vi "队列采集速度.vi"() -> ()   [LabVIEW 2019, in "test.lvlib"]
uses:
  SubVI/test.lvlib
  SubVI/config.ctl
  <vilib>/NI/Modbus Library/API/Master/Modbus Master.lvclass
  SubVI/Instrument.ctl
  lib/QDInstrument.dll
panel:
  out "元素":T1={"initialize"="", "6221"={"6221 Resource"="GPIB0::24::INSTR", "Delta status"=FALSE}, "7001"={"Ch"=FALSE}, "SR830+6221"={"source"=0, "阻抗"=0.0, "量程入 4"=0, "量程入 3"=0, "量程入 2"=0, "量程入 1"=0, "电流"=0.0, "SR830 2"=FALSE, "SR830 3"=FALSE, "SR830 4"=FALSE, "SR830 1"=FALSE, "VISA 1"="", "VISA 2"="", "VISA 3"="", "VISA 4"="", "量程"=enum."量程每次测量会判定"}, "2400"={"2400"=FALSE, "VISA"=""}, "ch"={"ch str"="", "ch1"=FALSE, "ch2"=FALSE, "布尔"=FALSE}, "error"=FALSE, "数据文件路径"=path "", "log"={"log路径"=path "", "log interval"=0.0}, "Instrument"={"335 Resource"="GPIB0::24::INSTR", "Input (0:A)"=0, "Instrument Type"=3, "quantum design"=refnum, "Heater Output (1:1)"=1, "335state"=refnum, "semaphore"=refnum, "TCP master instance"=refnum}} {"Instrument"."Input (0:A)" items=["A", "B"]; "Instrument"."Instrument Type" items=["PPMS", "VersaLab", "DynaCool", "SVSM", "Lakeshore335", "PPMS-Rotate"]; "Instrument"."Heater Output (1:1)" items=["1"=1, "2"=2]; "SR830+6221"."source" items=["SR830 1", "SR830 2", "SR830 3", "SR830 4"]}
  out "簇":T1={"initialize"="", "6221"={"6221 Resource"="GPIB0::24::INSTR", "Delta status"=FALSE}, "7001"={"Ch"=FALSE}, "SR830+6221"={"source"=0, "阻抗"=0.0, "量程入 4"=0, "量程入 3"=0, "量程入 2"=0, "量程入 1"=0, "电流"=0.0, "SR830 2"=FALSE, "SR830 3"=FALSE, "SR830 4"=FALSE, "SR830 1"=FALSE, "VISA 1"="", "VISA 2"="", "VISA 3"="", "VISA 4"="", "量程"=enum."量程每次测量会判定"}, "2400"={"2400"=FALSE, "VISA"=""}, "ch"={"ch str"="", "ch1"=FALSE, "ch2"=FALSE, "布尔"=FALSE}, "error"=FALSE, "数据文件路径"=path "", "log"={"log路径"=path "", "log interval"=0.0}, "Instrument"={"335 Resource"="GPIB0::24::INSTR", "Input (0:A)"=0, "Instrument Type"=3, "quantum design"=refnum, "Heater Output (1:1)"=1, "335state"=refnum, "semaphore"=refnum, "TCP master instance"=refnum}} {"Instrument"."Input (0:A)" items=["A", "B"]; "Instrument"."Instrument Type" items=["PPMS", "VersaLab", "DynaCool", "SVSM", "Lakeshore335", "PPMS-Rotate"]; "Instrument"."Heater Output (1:1)" items=["1"=1, "2"=2]; "SR830+6221"."source" items=["SR830 1", "SR830 2", "SR830 3", "SR830 4"]}
  out "当前时间 4":timestamp
  out "数值 4":i32
  out "当前时间 3":timestamp
  out "数值 3":i32
  out "当前时间 2":timestamp
  out "数值 2":i32
  out "数值":i32
  out "当前时间":timestamp
  # "(真是通道1，假是通道2)"
  # "(真是通道1，假是通道2)"
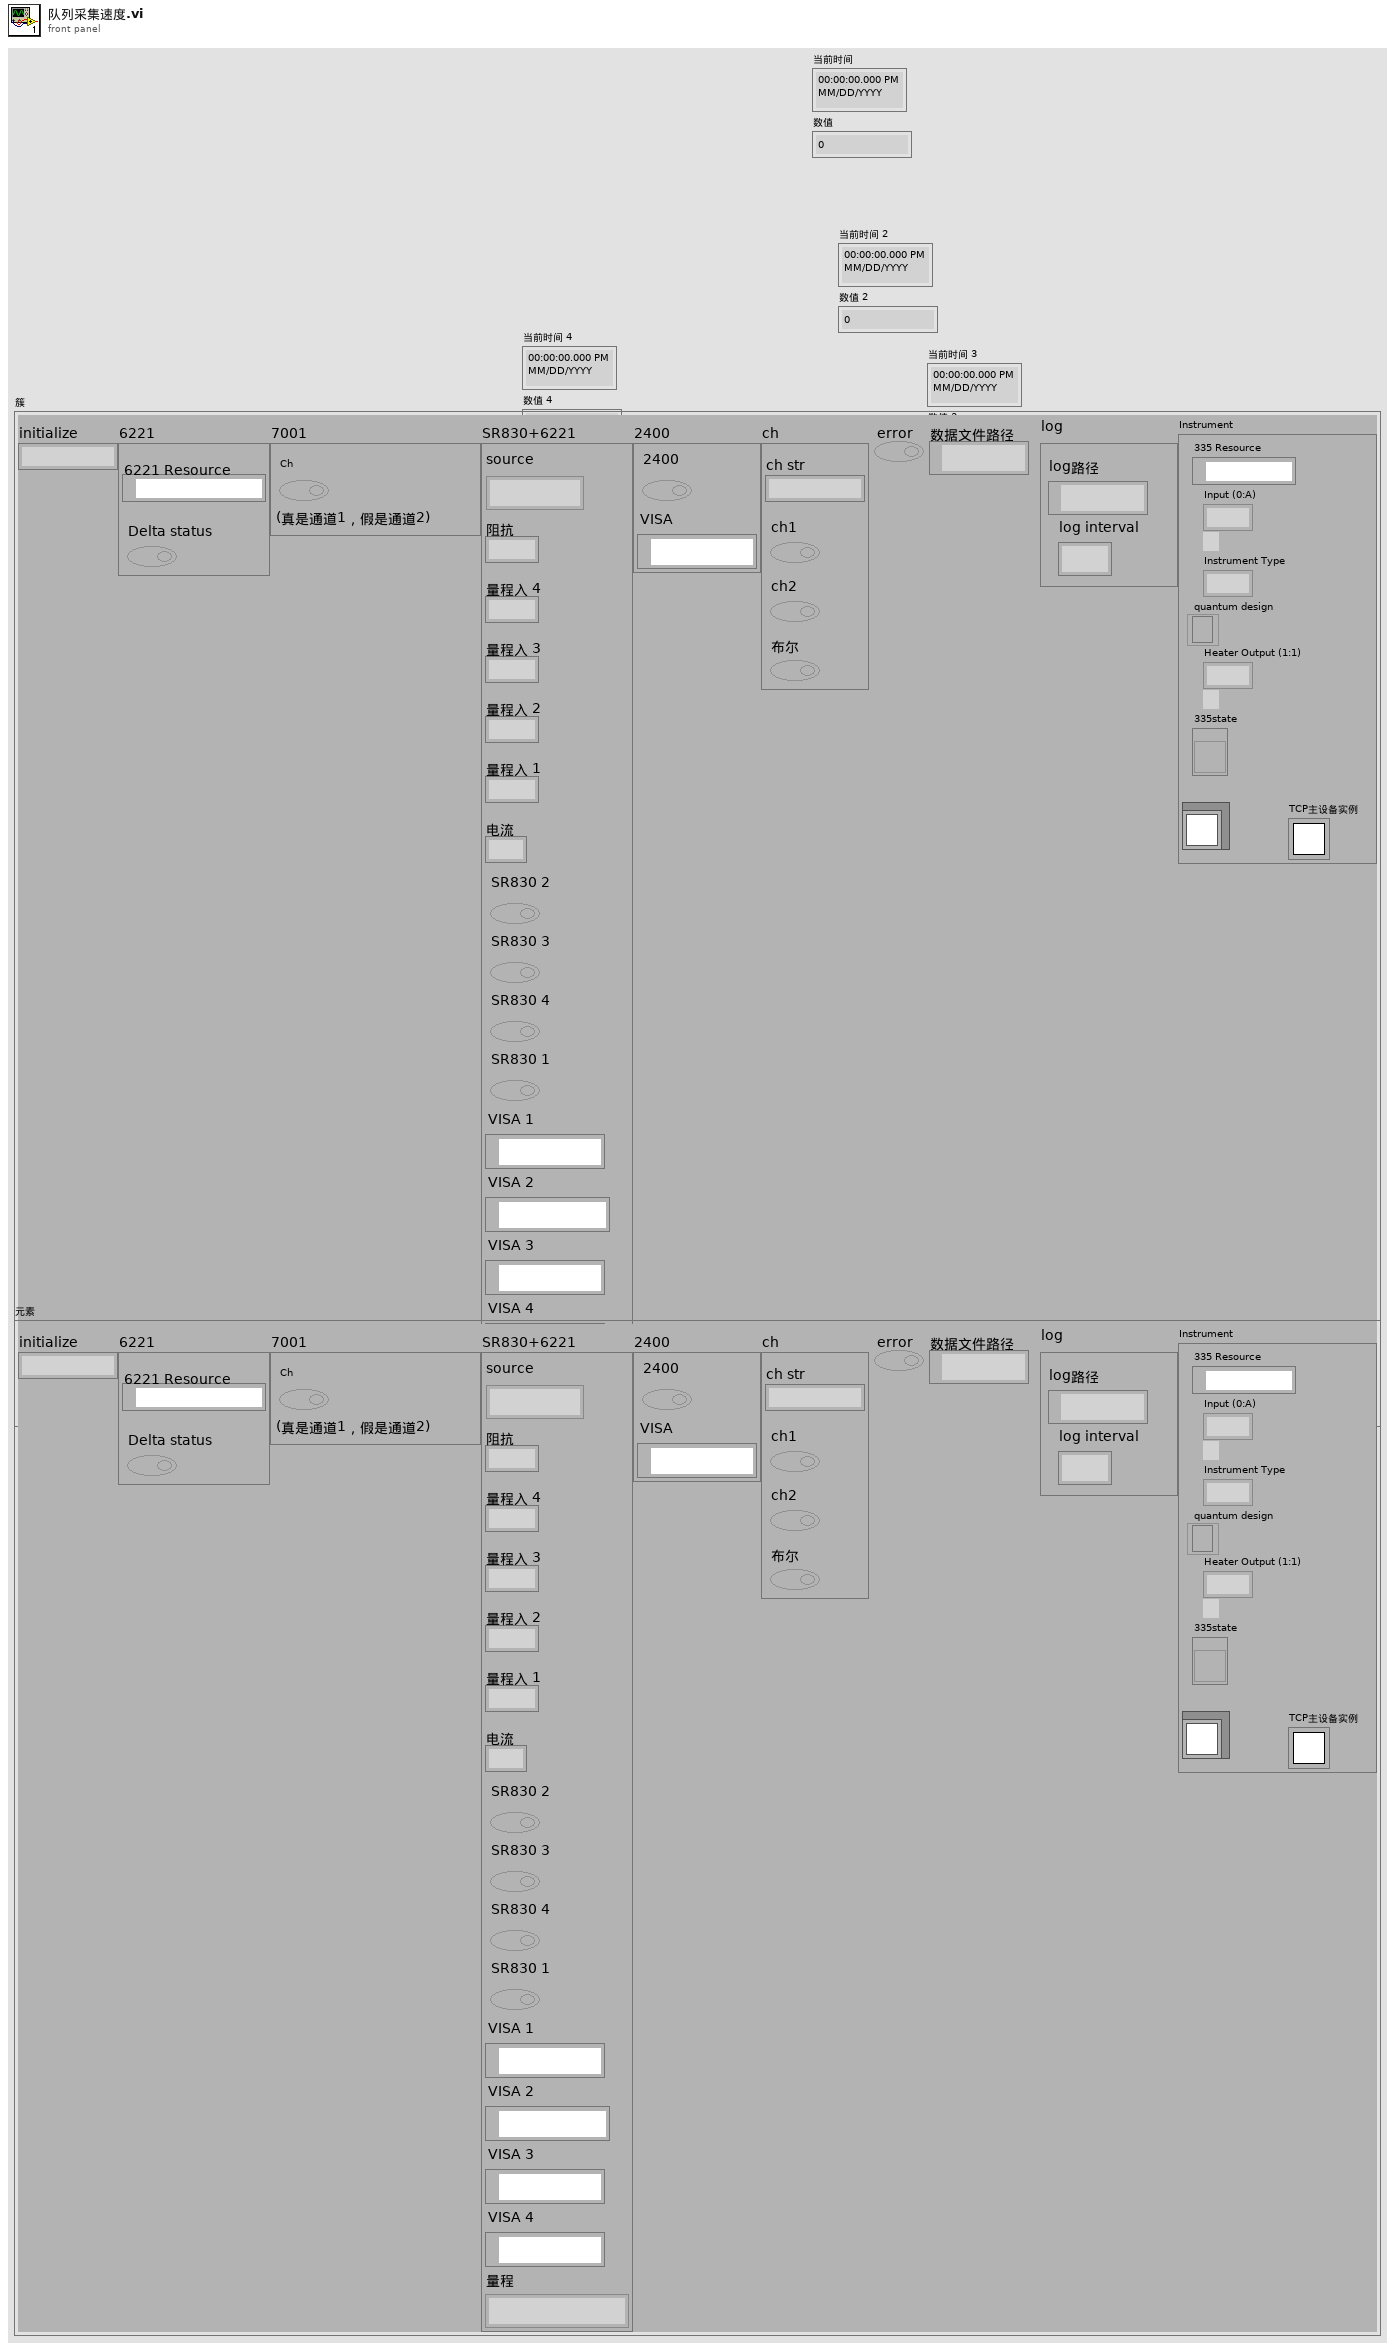
[diagram p1: front panel]
types:
  T1 = typedef "config.ctl" = cluster{"initialize":string, "6221":cluster{"6221 Resource":refnum<visa-resource-name>, "Delta status":bool}, "7001":cluster{"Ch":bool}, "SR830+6221":cluster{"source":u16, "阻抗":dbl, "量程入 4":i32, "量程入 3":i32, "量程入 2":i32, "量程入 1":i32, "电流":dbl, "SR830 2":bool, "SR830 3":bool, "SR830 4":bool, "SR830 1":bool, "VISA 1":refnum<visa-resource-name>, "VISA 2":refnum<visa-resource-name>, "VISA 3":refnum<visa-resource-name>, "VISA 4":refnum<visa-resource-name>, "量程":enum16{"量程每次测量会判定", "量程不变为设定值"}}, "2400":cluster{"2400":bool, "VISA":refnum<visa-resource-name>}, "ch":cluster{"ch str":string, "ch1":bool, "ch2":bool, "布尔":bool}, "error":bool, "数据文件路径":path, "log":cluster{"log路径":path, "log interval":dbl}, "Instrument":T2}
  T2 = typedef "Instrument.ctl" = cluster{"335 Resource":refnum<visa-resource-name>, "Input (0:A)":u16, "Instrument Type":i32, "quantum design":refnum<k24>, "Heater Output (1:1)":u16, "335state":refnum<vi>, "semaphore":T3, "TCP master instance":refnum<class "Modbus Master.lvclass">}
  T3 = typedef "Semaphore RefNum" = refnum<k1>
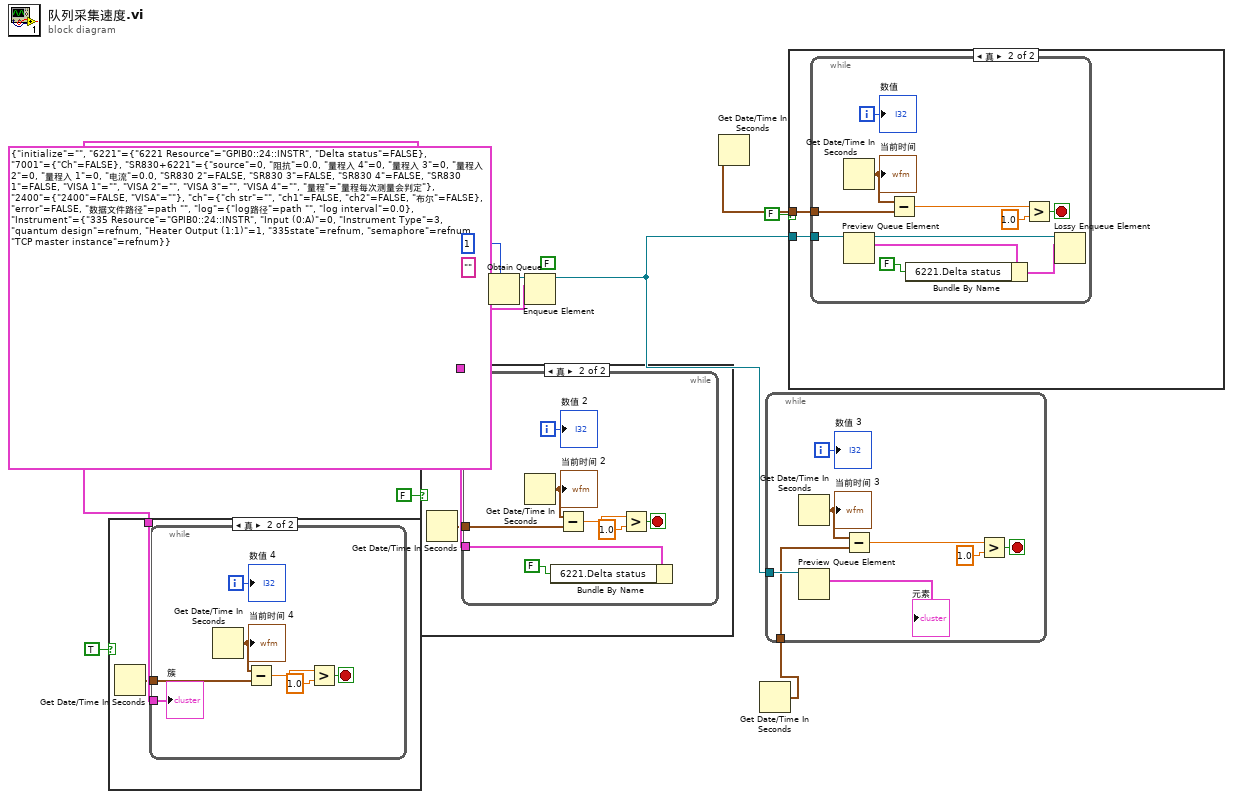
[diagram p0: block diagram]
diagram:
  (unwired) FALSE
  w1 = T1 {"initialize"="", "6221"={"6221 Resource"="GPIB0::24::INSTR", "Delta status"=FALSE}, "7001"={"Ch"=FALSE}, "SR830+6221"={"source"=0, "阻抗"=0.0, "量程入 4"=0, "量程入 3"=0, "量程入 2"=0, "量程入 1"=0, "电流"=0.0, "SR830 2"=FALSE, "SR830 3"=FALSE, "SR830 4"=FALSE, "SR830 1"=FALSE, "VISA 1"="", "VISA 2"="", "VISA 3"="", "VISA 4"="", "量程"=enum."量程每次测量会判定"}, "2400"={"2400"=FALSE, "VISA"=""}, "ch"={"ch str"="", "ch1"=FALSE, "ch2"=FALSE, "布尔"=FALSE}, "error"=FALSE, "数据文件路径"=path "", "log"={"log路径"=path "", "log interval"=0.0}, "Instrument"={"335 Resource"="GPIB0::24::INSTR", "Input (0:A)"=0, "Instrument Type"=3, "quantum design"=refnum, "Heater Output (1:1)"=1, "335state"=refnum, "semaphore"=refnum, "TCP master instance"=refnum}} ("簇")
  n1 = case shown="真" TRUE {
    tunnel: w1 -> [_ w12]
    frame False {
    }
    frame True {
      n2 = Get Date/Time In Seconds() -> (seconds since 1Jan1904=w11:timestamp)
      n3 = while {
        tunnel: w11 -> [w17]
        tunnel: w12 -> [w13]
        i -> [w18]
        stop <- w14 stop-if-true
        n4 = Get Date/Time In Seconds() -> (seconds since 1Jan1904=w19:timestamp)
        "当前时间 4" <- w19
        n5 = Subtract(x=w19, y=w17) -> (x-y=w16:dbl)
        n6 = Greater?(x=w16, y=1.0) -> (0:w14:bool)
        "数值 4" <- w18
        "簇" <- w13
      }
    }
  }
  n7 = case shown="真" FALSE {
    tunnel: w1 -> [_ w21]
    frame False {
    }
    frame True {
      n8 = Get Date/Time In Seconds() -> (seconds since 1Jan1904=w20:timestamp)
      n9 = while {
        tunnel: w20 -> [w26]
        tunnel: w21 -> [w22]
        i -> [w28]
        stop <- w23 stop-if-true
        n10 = Get Date/Time In Seconds() -> (seconds since 1Jan1904=w29:timestamp)
        "当前时间 2" <- w29
        n11 = Bundle By Name(cluster=w22, "6221.Delta status"=FALSE) -> ()  [unwired: 1 out]
        n12 = Subtract(x=w29, y=w26) -> (x-y=w25:dbl)
        n13 = Greater?(x=w25, y=1.0) -> (0:w23:bool)
        "数值 2" <- w28
      }
    }
  }
  n14 = Obtain Queue(max queue size (-1, unlimited)=1 ("队列最大值（-1，无限）"), name (unnamed)="" ("名称（未命名）"), element data type=w1) -> (queue out=w9:refnum<queue>)  [unwired: 2 in, 2 out]
  n15 = Enqueue Element(queue=w9, element=w1) -> (queue out=w6:refnum<queue>)  [unwired: 2 in, 2 out]
  n16 = Get Date/Time In Seconds() -> (seconds since 1Jan1904=w7:timestamp)
  n17 = Get Date/Time In Seconds() -> (seconds since 1Jan1904=w3:timestamp)
  n18 = while {
    tunnel: w6 -> [w37]
    tunnel: w3 -> [w30]
    i -> [w35]
    stop <- w31 stop-if-true
    n19 = Get Date/Time In Seconds() -> (seconds since 1Jan1904=w36:timestamp)
    "当前时间 3" <- w36
    n20 = Preview Queue Element(queue=w37) -> (element=→"元素":T1)  [unwired: 2 in, 3 out]
    n21 = Subtract(x=w36, y=w30) -> (x-y=w33:dbl)
    n22 = Greater?(x=w33, y=1.0) -> (0:w31:bool)
    "数值 3" <- w35
  }
  n23 = case shown="真" FALSE {
    tunnel: w7 -> [_ w39]
    tunnel: w6 -> [_ w38]
    frame False {
    }
    frame True {
      n24 = while {
        tunnel: w38 -> [w50]
        tunnel: w39 -> [w43]
        i -> [w48]
        stop <- w40 stop-if-true
        n25 = Get Date/Time In Seconds() -> (seconds since 1Jan1904=w49:timestamp)
        "当前时间" <- w49
        n26 = Preview Queue Element(queue=w50) -> (queue out=w45:refnum<queue>, element=w47:T1)  [unwired: 2 in, 2 out]
        n27 = Subtract(x=w49, y=w43) -> (x-y=w42:dbl)
        n28 = Bundle By Name(cluster=w47, "6221.Delta status"=FALSE) -> (w44:T1)
        n29 = Greater?(x=w42, y=1.0) -> (0:w40:bool)
        n30 = Lossy Enqueue Element(queue=w45, element=w44) -> ()  [unwired: 1 in, 4 out]
        "数值" <- w48
      }
    }
  }
